vi "AlliGator VIs Collection.vi"   [LabVIEW 2021]
uses:
  Action Engine/AlliGator Action Engine.lvlib
  GUI/AlliGator GUI.lvlib
  Settings/AlliGator Settings.lvlib
  Image Profile Window/AlliGator Image Profile Window.lvlib
  Graphs/Plot Editor/Plot Editor.lvlib
  Notebook/Notebook.lvlib
  Histograms/Histogram Window.lvlib
  Local Decay Window/AlliGator Local Decay Window.lvlib
  Palette/Palette.lvlib
  Phasor Plot Color Map/AlliGator Phasor Plot Color Map.lvlib
  ROIs/AlliGator ROIs.lvlib
  Dataset Information/AlliGator Dataset Information Window.lvlib
  Files/AlliGator Files.lvlib
  Phasor Harmonic/AlliGator Phasor Harmonics.lvlib
  Intensity Corrections/AlliGator Intensity Corrections.lvlib
  Decay Fit Parameter Map/AlliGator Decay Fit Parameter Map.lvlib
  Shot Noise Influence of Average Lifetime/AlliGator Shot Noise Influence on Average Lifetime.lvlib
  Fit Method Benchmark/AlliGator Fit Method Benchmark.lvlib
  Test Suites/AlliGator Test Suite.lvlib
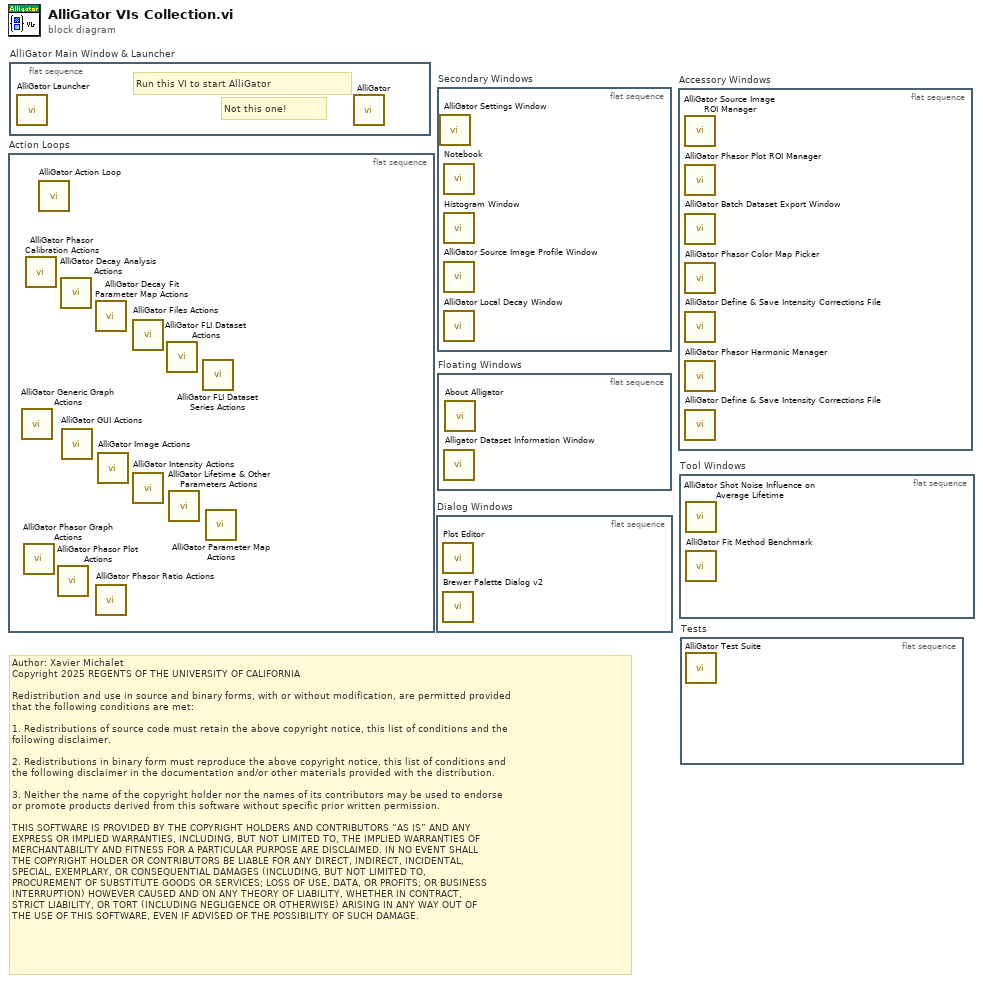
[diagram p0: block diagram]
diagram:
  # "Author: Xavier Michalet\nCopyright 2025 REGENTS OF THE UNIVERSITY OF CALIFORNIA\n\nRedistribution and use in source and binary forms, with or without modification, are permitted provided\nthat the following conditions are met:\n\n1. Redistributions of source code must retain the above copyright notice, this list of conditions and the\nfollowing disclaimer.\n\n2. Redistributions in binary form must reproduce the above copyright notice, this list of conditions and\nthe following disclaimer in the documentation and/or other materials provided with the distribution.\n\n3. Neither the name of the copyright holder nor the names of its contributors may be used to endorse \nor promote products derived from this software without specific prior written permission.\n\nTHIS SOFTWARE IS PROVIDED BY THE COPYRIGHT HOLDERS AND CONTRIBUTORS “AS IS” AND ANY \nEXPRESS OR IMPLIED WARRANTIES, INCLUDING, BUT NOT LIMITED TO, THE IMPLIED WARRANTIES OF\nMERCHANTABILITY AND FITNESS FOR A PARTICULAR PURPOSE ARE DISCLAIMED. IN NO EVENT SHALL\nTHE COPYRIGHT HOLDER OR CONTRIBUTORS BE LIABLE FOR ANY DIRECT, INDIRECT, INCIDENTAL, \nSPECIAL, EXEMPLARY, OR CONSEQUENTIAL DAMAGES (INCLUDING, BUT NOT LIMITED TO, \nPROCUREMENT OF SUBSTITUTE GOODS OR SERVICES; LOSS OF USE, DATA, OR PROFITS; OR BUSINESS\nINTERRUPTION) HOWEVER CAUSED AND ON ANY THEORY OF LIABILITY, WHETHER IN CONTRACT, \nSTRICT LIABILITY, OR TORT (INCLUDING NEGLIGENCE OR OTHERWISE) ARISING IN ANY WAY OUT OF\nTHE USE OF THIS SOFTWARE, EVEN IF ADVISED OF THE POSSIBILITY OF SUCH DAMAGE."
  n1 = flat-sequence "Action Loops" {
    frame #0 {
      n2 = call "AlliGator Generic Graph Actions.vi"() -> ()  [unwired: 11 in, 5 out]
      n3 = call "AlliGator Phasor Graph Actions.vi"() -> ()  [unwired: 11 in, 5 out]
      n4 = call "AlliGator Phasor Calibration Actions.vi"() -> ()  [unwired: 11 in, 5 out]
      n5 = call "AlliGator Action Loop.vi"() -> ()  [unwired: 11 in, 1 out]
      n6 = call "AlliGator Phasor Plot Actions.vi"() -> ()  [unwired: 11 in, 5 out]
      n7 = call "AlliGator Decay Analysis Actions.vi"() -> ()  [unwired: 11 in, 5 out]
      n8 = call "AlliGator GUI Actions.vi"() -> ()  [unwired: 10 in, 6 out]
      n9 = call "AlliGator Decay Fit Parameter Map Actions.vi"() -> ()  [unwired: 11 in, 5 out]
      n10 = call "AlliGator Phasor Ratio Actions.vi"() -> ()  [unwired: 11 in, 5 out]
      n11 = call "AlliGator Image Actions.vi"() -> ()  [unwired: 11 in, 5 out]
      n12 = call "AlliGator Files Actions.vi"() -> ()  [unwired: 11 in, 5 out]
      n13 = call "AlliGator Intensity Actions.vi"() -> ()  [unwired: 11 in, 5 out]
      n14 = call "AlliGator FLI Dataset Actions.vi"() -> ()  [unwired: 11 in, 5 out]
      n15 = call "AlliGator Lifetime & Other Parameters Actions.vi"() -> ()  [unwired: 11 in, 5 out]
      n16 = call "AlliGator FLI Dataset Series Actions.vi"() -> ()  [unwired: 11 in, 5 out]
      n17 = call "AlliGator Parameter Map Actions.vi"() -> ()  [unwired: 11 in, 5 out]
    }
  }
  n18 = flat-sequence "AlliGator Main Window & Launcher" {
    frame #0 {
      # "Not this one!"
      # "Run this VI to start AlliGator"
      n19 = call "AlliGator Launcher.vi"() -> ()  [unwired: 12 in]
      n20 = call "AlliGator.vi"() -> ()  [unwired: 1 in]
    }
  }
  n21 = flat-sequence "Dialog Windows" {
    frame #0 {
      n22 = call "Plot Editor.vi"() -> ()  [unwired: 9 in, 3 out]
      n23 = call "Brewer Palette Dialog v2.vi"() -> ()  [unwired: 7 in, 5 out]
    }
  }
  n24 = flat-sequence "Secondary Windows" {
    frame #0 {
      n25 = call "AlliGator Settings Window.vi"() -> ()  [unwired: 12 in]
      n26 = call "Notebook.vi"() -> ()  [unwired: 12 in]
      n27 = call "Histogram Window.vi"() -> ()  [unwired: 12 in]
      n28 = call "AlliGator Source Image Profile Window.vi"() -> ()  [unwired: 12 in]
      n29 = call "AlliGator Local Decay Window.vi"() -> ()  [unwired: 12 in]
    }
  }
  n30 = flat-sequence "Floating Windows" {
    frame #0 {
      n31 = call "Alligator Dataset Information Window.vi"() -> ()  [unwired: 12 in]
      n32 = call "About Alligator.vi"() -> ()  [unwired: 12 in]
    }
  }
  n33 = flat-sequence "Accessory Windows" {
    frame #0 {
      n34 = call "AlliGator Source Image ROI Manager.vi"() -> ()  [unwired: 12 in]
      n35 = call "AlliGator Phasor Plot ROI Manager.vi"() -> ()  [unwired: 12 in]
      n36 = call "AlliGator Batch Dataset Export Window.vi"() -> ()  [unwired: 12 in]
      n37 = call "AlliGator Phasor Color Map Picker.vi"() -> ()  [unwired: 12 in]
      n38 = call "AlliGator Define & Save Intensity Corrections File.vi"() -> ()  [unwired: 12 in]
      n39 = call "AlliGator Phasor Harmonic Manager.vi"() -> ()  [unwired: 12 in]
      n40 = call "AlliGator Define & Save Intensity Corrections File.vi"() -> ()  [unwired: 12 in]
    }
  }
  n41 = flat-sequence "Tool Windows" {
    frame #0 {
      n42 = call "AlliGator Shot Noise Influence on Average Lifetime.vi"() -> ()  [unwired: 12 in]
      n43 = call "AlliGator Fit Method Benchmark.vi"() -> ()  [unwired: 12 in]
    }
  }
  n44 = flat-sequence "Tests" {
    frame #0 {
      n45 = call "AlliGator Test Suite.vi"() -> ()  [unwired: 12 in]
    }
  }
